vi "dfd_Build Filter Bank Spec XML String.vi"(8 "error in (no error)":errorcluster, 11 "filter bank":T1 {"mFBank_SynthesisFilters"."mMRate_SumWl" min=1 max=32 step=1; "mFBank_SynthesisFilters"."mMRate_InputIwl" min=1 max=32 step=1; "mFBank_SynthesisFilters"."mMRate_GainWl" min=1 max=32 step=1; "mFBank_SynthesisFilters"."mMRate_OutputWl" min=1 max=32 step=1; "mFBank_SynthesisFilters"."mMRate_InputWl" min=1 max=32 step=1; "mFBank_SynthesisFilters"."mMRate_CoefWl" min=1 max=32 step=1; "mFBank_SynthesisFilters"."mMRate_Mode" items=["Default"=-1, "No Rate Change"=0, "Interpolation"=1, "Decimation"=2, "Interpolated"=3, "Rational"=4]; "mFBank_AnalysisFilters"."mMRate_SumWl" min=1 max=32 step=1; "mFBank_AnalysisFilters"."mMRate_InputIwl" min=1 max=32 step=1; "mFBank_AnalysisFilters"."mMRate_GainWl" min=1 max=32 step=1; "mFBank_AnalysisFilters"."mMRate_OutputWl" min=1 max=32 step=1; "mFBank_AnalysisFilters"."mMRate_InputWl" min=1 max=32 step=1; "mFBank_AnalysisFilters"."mMRate_CoefWl" min=1 max=32 step=1; "mFBank_AnalysisFilters"."mMRate_Mode" items=["Default"=-1, "No Rate Change"=0, "Interpolation"=1, "Decimation"=2, "Interpolated"=3, "Rational"=4]; "mFBank_Type" items=["Uniform", "Non-Uniform"]}) -> (0 "error out":errorcluster, 2 "String":string, 3 "dup filter bank":T1 {"mFBank_SynthesisFilters"."mMRate_SumWl" min=1 max=32 step=1; "mFBank_SynthesisFilters"."mMRate_InputIwl" min=1 max=32 step=1; "mFBank_SynthesisFilters"."mMRate_GainWl" min=1 max=32 step=1; "mFBank_SynthesisFilters"."mMRate_OutputWl" min=1 max=32 step=1; "mFBank_SynthesisFilters"."mMRate_InputWl" min=1 max=32 step=1; "mFBank_SynthesisFilters"."mMRate_CoefWl" min=1 max=32 step=1; "mFBank_SynthesisFilters"."mMRate_Mode" items=["Default"=-1, "No Rate Change"=0, "Interpolation"=1, "Decimation"=2, "Interpolated"=3, "Rational"=4]; "mFBank_AnalysisFilters"."mMRate_SumWl" min=1 max=32 step=1; "mFBank_AnalysisFilters"."mMRate_InputIwl" min=1 max=32 step=1; "mFBank_AnalysisFilters"."mMRate_GainWl" min=1 max=32 step=1; "mFBank_AnalysisFilters"."mMRate_OutputWl" min=1 max=32 step=1; "mFBank_AnalysisFilters"."mMRate_InputWl" min=1 max=32 step=1; "mFBank_AnalysisFilters"."mMRate_CoefWl" min=1 max=32 step=1; "mFBank_AnalysisFilters"."mMRate_Mode" items=["Default"=-1, "No Rate Change"=0, "Interpolation"=1, "Decimation"=2, "Interpolated"=3, "Rational"=4]; "mFBank_Type" items=["Uniform", "Non-Uniform"]})   [LabVIEW 2017, in "NI_DigFilter_FilterBank.lvlib"]
uses:
  <vilib>/addons/Digital Filter Design/NI_DigFilter_FilterBank.lvlib
  <vilib>/addons/Digital Filter Design/FilterBank.llb/Object/DFD Filter Bank Obj.ctl
  <vilib>/addons/Digital Filter Design/_Objects.llb/DFD Multirate Filter Obj.ctl
  <vilib>/addons/Digital Filter Design/_Objects.llb/DFD Multirate Mode.ctl
  <vilib>/addons/Digital Filter Design/_Objects.llb/DFD Coef Norm Type.ctl
  <vilib>/addons/Digital Filter Design/_Objects.llb/DFD Round-off Mode.ctl
  <vilib>/addons/Digital Filter Design/_Objects.llb/DFD FXP MRate Multiply Mode.ctl
  <vilib>/addons/Digital Filter Design/FilterBank.llb/Object/DFD Filter Bank Processing Method.ctl
  <vilib>/addons/Digital Filter Design/FilterBank.llb/Object/DFD Filter Bank Type.ctl
  <vilib>/addons/Digital Filter Design/NI_DigFilter_Process.lvlib
  <vilib>/addons/Digital Filter Design/NI_DigFilterLicensed.lvlib
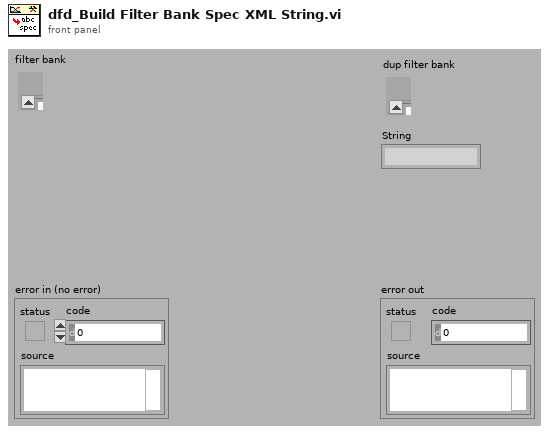
[diagram p1: front panel]
types:
  T1 = typedef "NI_DigFilter_FilterBank.lvlib/DFD Filter Bank Obj.ctl" = cluster{"mFBank_AnalysisFilters":T2[], "mFBank_SynthesisFilters":T2[], "mFBank_#Bands":i32, "mFBank_ProcMethod":T7, "mFBank_Coeffs":dbl[], "mFBank_Gain":dbl, "mFBank_Delay":i32, "mFBank_Type":T8}
  T2 = typedef "NI_DigFilterLicensed.lvlib/DFD Multirate Filter Obj.ctl" = cluster{"mMRate_Structure":enum16{"CIC", "FIR", "IIR", "Lattice"}, "mMRate_Mode":T3, "mMRate_Factor":i32, "mMRate_FIRParams":cluster{"mMRate_FIR_H":dbl[], "mMRate_FIR_IsNyquist?":bool, "mMRate_FIR_IsSymmetric?":bool}, "mMRate_CICParams":cluster{"mMRate_CIC_#Stage":i32, "mMRate_CIC_Lag":i32, "mMRate_CIC_Type":enum16{"Lowpass", "Highpass"}}, "mMRate_Order":i32, "mMRate_Version":string, "mMRate_Comments":string, "mMRate_RationalFactor":cluster{"mMRate_L":i32, "mMRate_M":i32}, "mMRate_Fs":dbl, "mMRate_Quantized?":bool, "mMRate_QFilterGain":dbl, "mMRate_CoefWl":i16, "mMRate_Scaling":cluster{"mMRate_ScaleByPowerOf2?":bool, "mMRate_ScaleType":T4}, "mMRate_InputWl":i16, "mMRate_OutputWl":i16, "mMRate_OutputMode":T5, "mMRate_MultMode":T6, "mMRate_BitPruning":bool, "mMRate_GainWl":i16, "mMRate_OutputFwl":i16, "mMRate_SumIwl":i16, "mMRate_InputIwl ":i16, "mMRate_SumWl":i16, "mMRate_CoefIwl":i16}
  T3 = typedef "NI_DigFilterLicensed.lvlib/DFD Multirate Mode.ctl" = i16
  T4 = typedef "NI_DigFilterLicensed.lvlib/DFD Coef Norm Type.ctl" = enum16{"No Norm", "Time Domain 1-Norm", "Time Domain 2-Norm", "Time Domain Inf-Norm"}
  T5 = typedef "NI_DigFilterLicensed.lvlib/DFD Round-off Mode.ctl" = enum16{"Nearest", "Truncation"}
  T6 = typedef "NI_DigFilterLicensed.lvlib/DFD FXP MRate Multiply Mode.ctl" = enum16{"Truncated", "Full"}
  T7 = typedef "NI_DigFilter_FilterBank.lvlib/DFD Filter Bank Processing Method.ctl" = enum16{"General", "2-Band QMF Lattice", "Cosine-Modulated"}
  T8 = typedef "NI_DigFilter_FilterBank.lvlib/DFD Filter Bank Type.ctl" = u16
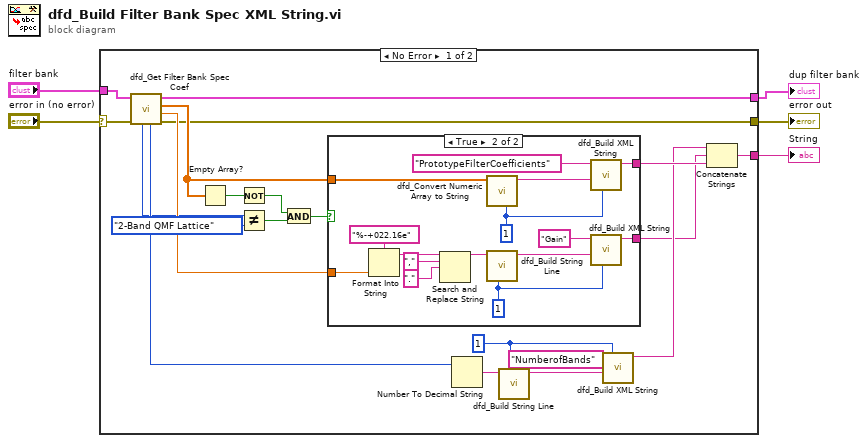
[diagram p0: block diagram]
diagram:
  n1 = case shown="No Error" "error in (no error)" {
    selector: "error in (no error)" -> [w12 w43]
    tunnel: [w26 _] -> w5
    tunnel: "filter bank" -> [w20 w42]
    tunnel: [w14 w43] -> w3
    tunnel: [w13 w42] -> w2
    frame No Error {
      w18 = 1 ("indent order")
      n2 = call <vilib>:"dfd_Get Filter Bank Spec Coef.vi"("error in (no error)"=w12, "filter bank"=w20) -> ("error out"=w14:errorcluster, "gain"=w16:dbl, "coefficients"=w17:dbl[], "dup filter bank"=w13:T1, "number of bands"=w19:i32, "processing method"=w11:T7)  [unwired: 4 in]
      n3 = Empty Array?(array=w17) -> (empty?=w9:bool)
      n4 = Not(x=w9) -> (.not. x?=w7:bool)
      n5 = Not Equal?(x=w11, y=DFD_Filter_Bank_Processing_Method."2-Band QMF Lattice") -> (x != y?=w6:bool)
      n6 = And(x=w7, y=w6) -> (x .and. y?=w8:bool)
      n7 = case shown="True" w8 {
        tunnel: w17 -> [_ w38]
        tunnel: [_ w37] -> w25
        tunnel: w16 -> [_ w29]
        tunnel: [_ w27] -> w15
        frame False {
        }
        frame True {
          w28 = 1 ("indent order")
          w39 = 1 ("indent order")
          n8 = Format Into String(format string="%-+022.16e", w29) -> (resulting string=w32:string)  [unwired: 2 in, 1 out]
          n9 = Search and Replace String(input string=w32, search string=",", replace string="." ("replace string (\"\")")) -> (result string=w33:string)  [unwired: 2 in, 6 out]
          n10 = call <vilib>:"dfd_Convert Numeric Array to String.vi"("indent order"=w39, "numeric array"=w38) -> ("string"=w41:string)  [unwired: 4 in, 5 out]
          n11 = call <vilib>:"dfd_Build String Line.vi"("indent order"=w28, "string"=w33) -> ("string line"=w36:string)  [unwired: 9 out]
          n12 = call <vilib>:"dfd_Build XML String.vi"("indent order"=w39, "string in"=w41, "element name"="PrototypeFilterCoefficients") -> ("xml string out"=w37:string)  [unwired: 2 in, 6 out]
          n13 = call <vilib>:"dfd_Build XML String.vi"("indent order"=w28, "string in"=w36, "element name"="Gain") -> ("xml string out"=w27:string)  [unwired: 2 in, 6 out]
        }
      }
      n14 = Number To Decimal String(number=w19) -> (decimal integer string=w24:string)  [unwired: 1 in]
      n15 = call <vilib>:"dfd_Build String Line.vi"("indent order"=w18, "string"=w24) -> ("string line"=w23:string)  [unwired: 9 out]
      n16 = call <vilib>:"dfd_Build XML String.vi"("indent order"=w18, "string in"=w23, "element name"="NumberofBands") -> ("xml string out"=w21:string)  [unwired: 2 in, 6 out]
      n17 = Concatenate Strings(w21, w15, w25) -> (w26:string)
    }
    frame Error {
    }
  }
  "String" <- w5
  "error out" <- w3
  "dup filter bank" <- w2
